vi "GetToteTargetPos.vi"(1 "Pick up from Side":bool=TRUE, 2 "X Offset":dbl format="%#_13g", 3 "Angle (rad)":dbl format="%#_13g", 4 "Dist":dbl format="%#_13g") -> (0 "Target X/Y/a":cluster{dbl, dbl, dbl})   [LabVIEW 2014]
uses:
  Robot Global Data.vi
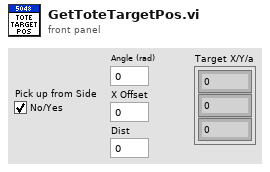
[diagram p1: front panel]
types:
  T1 = cluster{"X Position":dbl, "Y Position":dbl, "Angle":dbl}
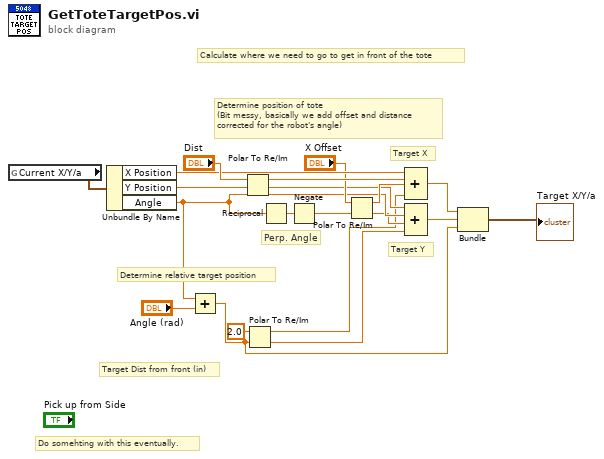
[diagram p0: block diagram]
diagram:
  # "Do somehting with this eventually."
  # "Determine relative target position"
  # "Target Y"
  # "Target X"
  # "Perp. Angle"
  # "Determine position of tote\n(Bit messy, basically we add offset and distance\ncorrected for the robot's angle)"
  # "Target Dist from front (in)"
  # "Calculate where we need to go to get in front of the tote"
  n1 = global read "Robot Global Data.vi" "Current X/Y/a"() -> (w20:T1)
  n2 = Unbundle By Name(w20) -> ("X Position"=w17:dbl, "Y Position"=w12:dbl, "Angle"=w7:dbl)
  n3 = Add(x=w7, y="Angle (rad)") -> (x+y=w2:dbl)
  n4 = Polar To Re/Im(2:w7, 3:"Dist") -> (0:w11:dbl, 1:w16:dbl)
  n5 = Polar To Re/Im(2:w2, 3:2.0 ("r")) -> (0:w5:dbl, 1:w6:dbl)
  n6 = Reciprocal(x=w7) -> (1/x=w18:dbl)
  n7 = Negate(x=w18) -> (-x=w15:dbl)
  n8 = Polar To Re/Im(2:w15, 3:"X Offset") -> (0:w10:dbl, 1:w13:dbl)
  n9 = Compound Arithmetic op=ADD(w17, w16, w13, w6) -> (w4:dbl)
  n10 = Compound Arithmetic op=ADD(w12, w11, w10, w5) -> (w3:dbl)
  n11 = Bundle(w4, w3, w2) -> (→"Target X/Y/a":cluster{dbl, dbl, dbl})  [unwired: 1 in]
